vi "Start.vi"(8 "error in (no error)":errorcluster, 11 "Study Base in":refnum<class "Study Base.lvclass">) -> (0 "error out":errorcluster, 3 "Study Base out":refnum<class "Study Base.lvclass">)   [LabVIEW 2023, in "HAL GOOP4.lvlib" / "Study Base.lvclass"]
uses:
  Study Base.lvclass
  Study Base.lvclass/Study Base.ctl
  Task Base/Call Perform Action.vi
  Task Base/Task Base.lvclass
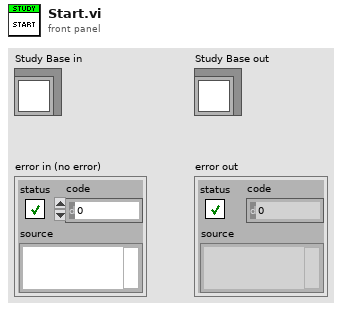
[diagram p1: front panel]
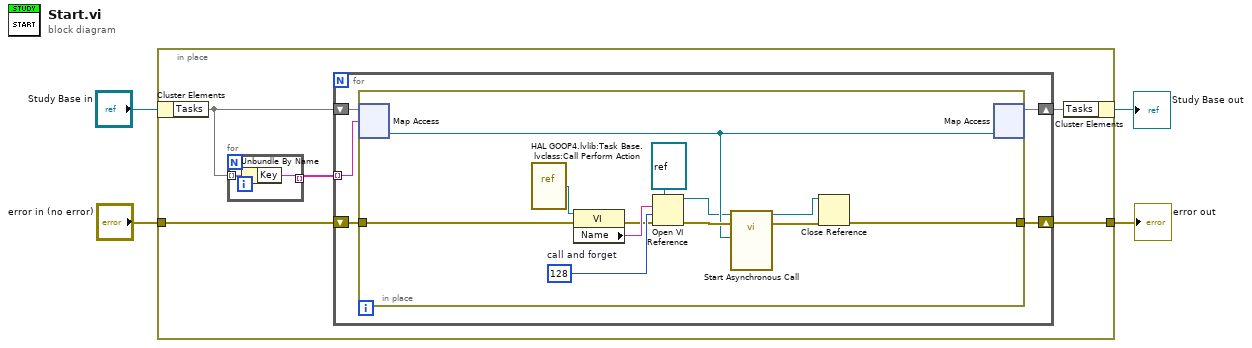
[diagram p0: block diagram]
diagram:
  n1 = in-place {
    in-place-border: "error in (no error)" -> [w5]
    in-place-border: [w9] -> w1
    n2 = in-place-cluster #1("Study Base in") -> ("Tasks"=w7:map{string, refnum<class "Task Base.lvclass">})
    n3 = for {
      tunnel: [w28] -> w8 mode=indexing
      tunnel: w7 -> [w27] mode=indexing
      n4 = Unbundle By Name(w27) -> ("Key"=w28:string)
    }
    n5 = for {
      tunnel: w8 -> [w12] mode=indexing
      shift-right: [w11] -> w6
      shift-left: w7 -> [w13]
      shift-right: [w14] -> w9
      shift-left: w5 -> [w10]
      n6 = in-place {
        in-place-border: [w23] -> w14
        in-place-border: w10 -> [w18]
        w25 = 128  # call and forget
        n7 = in-place-map #2(w13, w12) -> (w21:refnum<class "Task Base.lvclass">)  [unwired: 1 in, 1 out]
        n8 = vi-ref "HAL GOOP4.lvlib:Task Base.lvclass:Call Perform Action.vi"() -> (w20:refnum<vi>)
        n9 = property class="VI"(reference=w20, error in=w18) -> (error out=w17:errorcluster, "Name"=w19:string)  [unwired: 1 out]
        n10 = Open VI Reference(type specifier VI Refnum (for type only)=refnum<vi> refnum, vi path=w19, options=w25, error in (no error)=w17) -> (vi reference=w16:refnum<vi>, error out=w26:errorcluster)  [unwired: 2 in]
        n11 = call-by-ref "Start Asynchronous Call"(reference=w16, error in=w26, "Task Base in"=w21) -> (reference out=w22:refnum<vi>, error out=w24:errorcluster)  [unwired: 8 in, 3 out]
        n12 = Close Reference(reference=w22, error in (no error)=w24) -> (error out=w23:errorcluster)
        n13 = in-place-map #2(w21) -> (w11:map{string, refnum<class "Task Base.lvclass">})  [unwired: 1 in, 2 out]
      }
    }
    n14 = in-place-cluster #1("Tasks"=w6) -> (→"Study Base out":refnum<class "Study Base.lvclass">)
  }
  "error out" <- w1
